vi "Unflatten from JSON Config.vi"(8 "error in (no error)":errorcluster, 10 "JSON Text":string, 11 "Tag in":refnum<class "Tag.lvclass">) -> (0 "error out":errorcluster, 3 "Tag out":refnum<class "Tag.lvclass">)   [LabVIEW 2018, in "Tag Engine.lvlib" / "Tag.lvclass"]
doc: "_SubVI_"
uses:
  Tag.lvclass
  <vilib>/Utility/Data Type/Type Definitions/Data Type.ctl
  Tag.lvclass/Tag.ctl
  8616131f-fb1e-43f1-803b-b97b3369c86a.vi
  <vilib>/JDP Science/JSONtext/JSON text to Variant.vi
  Set Properties from Initial.vi
  <vilib>/JDP Science/JSONtext/LVClass Serializer/JSONtext LVClass Serializer.lvclass
  <vilib>/Utility/Data Type/NI_Data Type.lvlib
  <vilib>/JDP Science/JDP Science Common Utilities/Base64/Base64 Support.lvlib
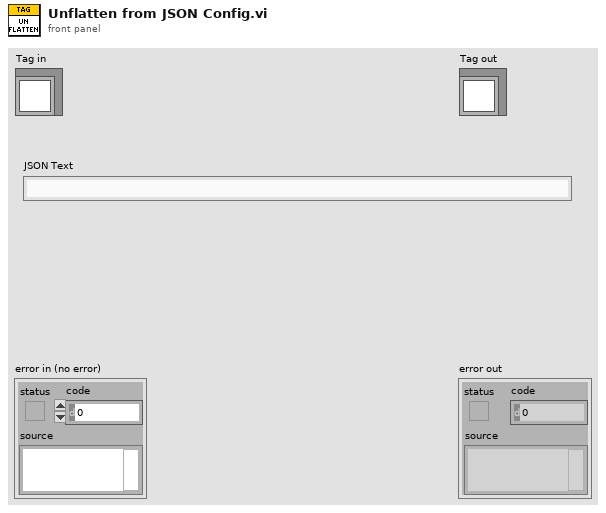
[diagram p1: front panel]
types:
  T1 = typedef "NI_Data Type.lvlib/Data Type.ctl" = enum8{"Invalid Type", "Void", "I8", "I16", "I32", "I64", "U8", "U16", "U32", "U64", "Single Float", "Double Float", "Extended Float", "Single Complex", "Double Complex", "Extended Complex", "Enum U8", "Enum U16", "Enum U32", "Enum U64", "Single Float With Unit", "Double Float With Unit", "Extended Float With Unit", "Single Complex with Unit", "Double Complex with Unit", "Extended Complex with Unit", "Boolean", "String", "Path", "Picture", "Tag", "Array", "Cluster", "Variant", "LV Variant", "Waveform", "Timestamp", "Digital Waveform", "Digital Data", "ExpressData", "Refnum", "External Data", "VI", "Poly VI", "LabVIEW Class Instance", "Fixed Point"}
  T2 = cluster{"name":string, "type":T1, "typeString":i16[], "properties":cluster{"name":string, "value":string, "typeString":i16[]}[]}
  T3 = cluster{"name":string, "value":string, "typeString":i16[]}[]
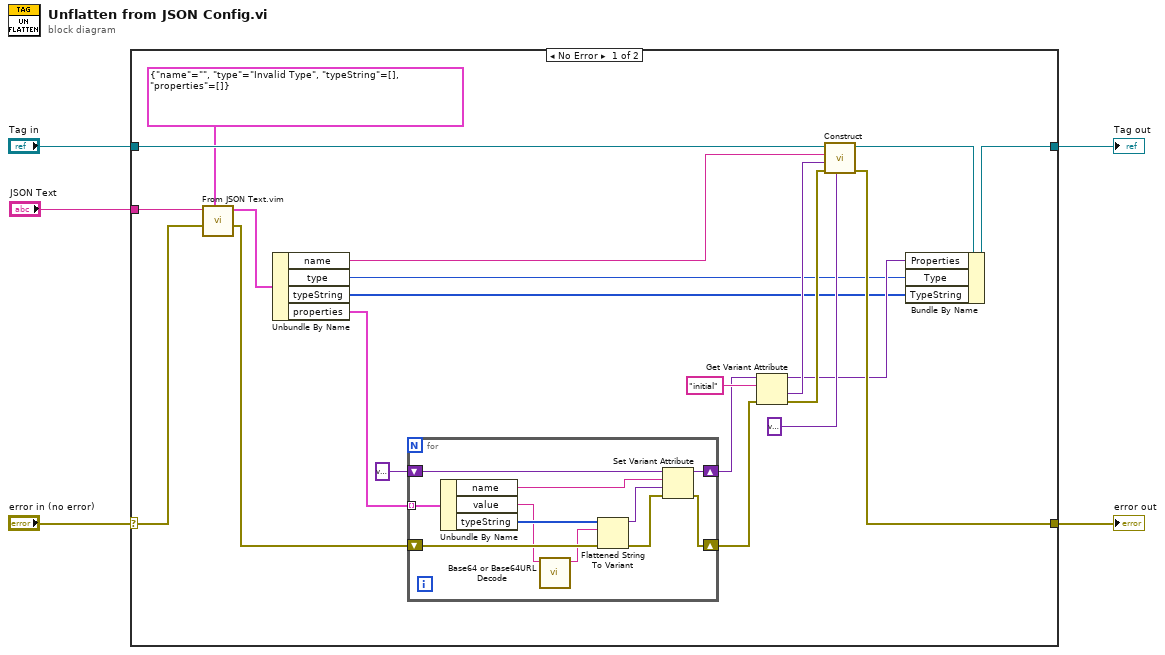
[diagram p0: block diagram]
diagram:
  n1 = case shown="No Error" "error in (no error)" {
    selector: "error in (no error)" -> [w15 w39]
    tunnel: [w25 w39] -> w4
    tunnel: [w19 w38] -> w2
    tunnel: "Tag in" -> [w26 w38]
    tunnel: "JSON Text" -> [w17 _]
    frame No Error {
      n2 = call "From JSON Text.vim"("Data Type and Default Value"=T2 {"name"="", "type"=enum."Invalid Type", "typeString"=[], "properties"=[]}, "error in (no error)"=w15, "JSON"=w17) -> ("error out"=w9:errorcluster, "Data out"=w14:T2)  [unwired: 7 in]
      n3 = Unbundle By Name(w14) -> ("name"=w13:string, "type"=w7:T1, "typeString"=w6:i16[], "properties"=w12:T3)
      n4 = for {
        tunnel: w12 -> [w37] mode=indexing
        shift-right: [w33] -> w10
        shift-left: variant -> [w32]
        shift-right: [w30] -> w8
        shift-left: w9 -> [w29]
        n5 = Unbundle By Name(w37) -> ("name"=w34:string, "value"=w28:string, "typeString"=w36:i16[])
        n6 = call <vilib>:"Base64 or Base64URL Decode.vi"("Base64 or Base64URL"=w28) -> ("Decoded"=w27:string)  [unwired: 10 in]
        n7 = Flattened String To Variant(4:w29, 6:w27, 7:w36) -> (0:w31:errorcluster, 3:w35:variant)
        n8 = Set Variant Attribute(Variant=w32, name=w34, value=w35, error in=w31) -> (Variant out=w33:variant, error out=w30:errorcluster)  [unwired: 1 out]
      }
      n9 = Get Variant Attribute(Variant=w10, name="initial", error in=w8) -> (duplicate Variant=w18:variant, value=w22:variant, error out=w23:errorcluster)  [unwired: 1 in, 1 out]
      n10 = call "Construct.vi"("Properties"=variant, "error in (no error)"=w23, "Initial Value"=w22, "Name"=w13, "Tag in"=w26) -> ("error out"=w25:errorcluster, "Tag out"=w20:refnum<class "Tag.lvclass">)  [unwired: 5 in]
      n11 = Bundle By Name(cluster=w20, "Properties"=w18, "Type"=w7, "TypeString"=w6) -> (w19:refnum<class "Tag.lvclass">)
    }
    frame Error {
    }
  }
  "error out" <- w4
  "Tag out" <- w2
